vi "Purge.vi"(5 "Digital I/O Pin":u8=7, 7 "Arduino Resource":T1={"VISA resource"="GlueCTRL", "Board Type"=enum."Uno", "Connection Type"=enum."USB / Serial", "Bytes Per Packet (15)"=15}, 9 "Axis Speeds":T3={"X [mm/s]"=25.0, "Y [mm/s]"=25.0, "Z [mm/s]"=10.0}, 10 "Start Position [mm]":dbl[](array[numeric]), 11 ".NET Refnum In":refnum<k24>) -> ()   [LabVIEW 2016]
uses:
  C:/Users/Aerotech/Documents/BNLStaveAssembly-blueprint/Bin/Aerotech.A3200.dll
  BNLStaveAssembly-blueprint/Bin/Aerotech.A3200.dll
  <vilib>/LabVIEW Interface for Arduino/Type Defs/Arduino Resource.ctl
  <vilib>/LabVIEW Interface for Arduino/Type Defs/Board Type.ctl
  <vilib>/LabVIEW Interface for Arduino/LabVIEW Interface for Arduino.lvlib
panel:
  in  "Absolute Purge Height [mm]":dbl=-30.0 format="%#_13g"
  in  "Relative Change in X, Y to Purge [mm]":dbl[](array[numeric])=[0.0, -50.0, 0.0]
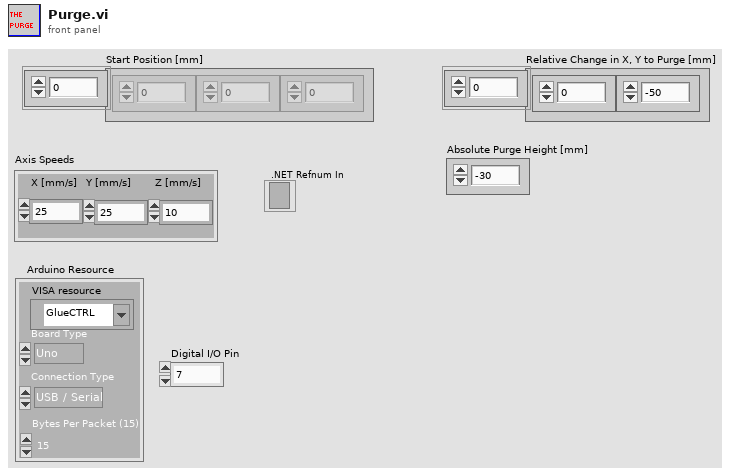
[diagram p1: front panel]
types:
  T1 = typedef "LabVIEW Interface for Arduino.lvlib/Arduino Resource.ctl" = cluster{"VISA resource":refnum<visa-resource-name>, "Board Type":T2, "Connection Type":enum8{"USB / Serial"}, "Bytes Per Packet (15)":u8}
  T2 = typedef "LabVIEW Interface for Arduino.lvlib/Board Type.ctl" = enum16{"Uno", "Dimuelanove w/Atmega 328", "Mega 2560"}
  T3 = cluster{"X [mm/s]":dbl, "Y [mm/s]":dbl, "Z [mm/s]":dbl}
  T4 = cluster{"Start Position [mm][0]":dbl, "Start Position [mm][1]":dbl, "Start Position [mm][2]":dbl}
  T5 = cluster{"Final X":dbl, "Final Y":dbl, "Final Z":dbl}
  T6 = cluster{"Final Position[0]":dbl, "Final Position[1]":dbl, "Final Position[2]":dbl}
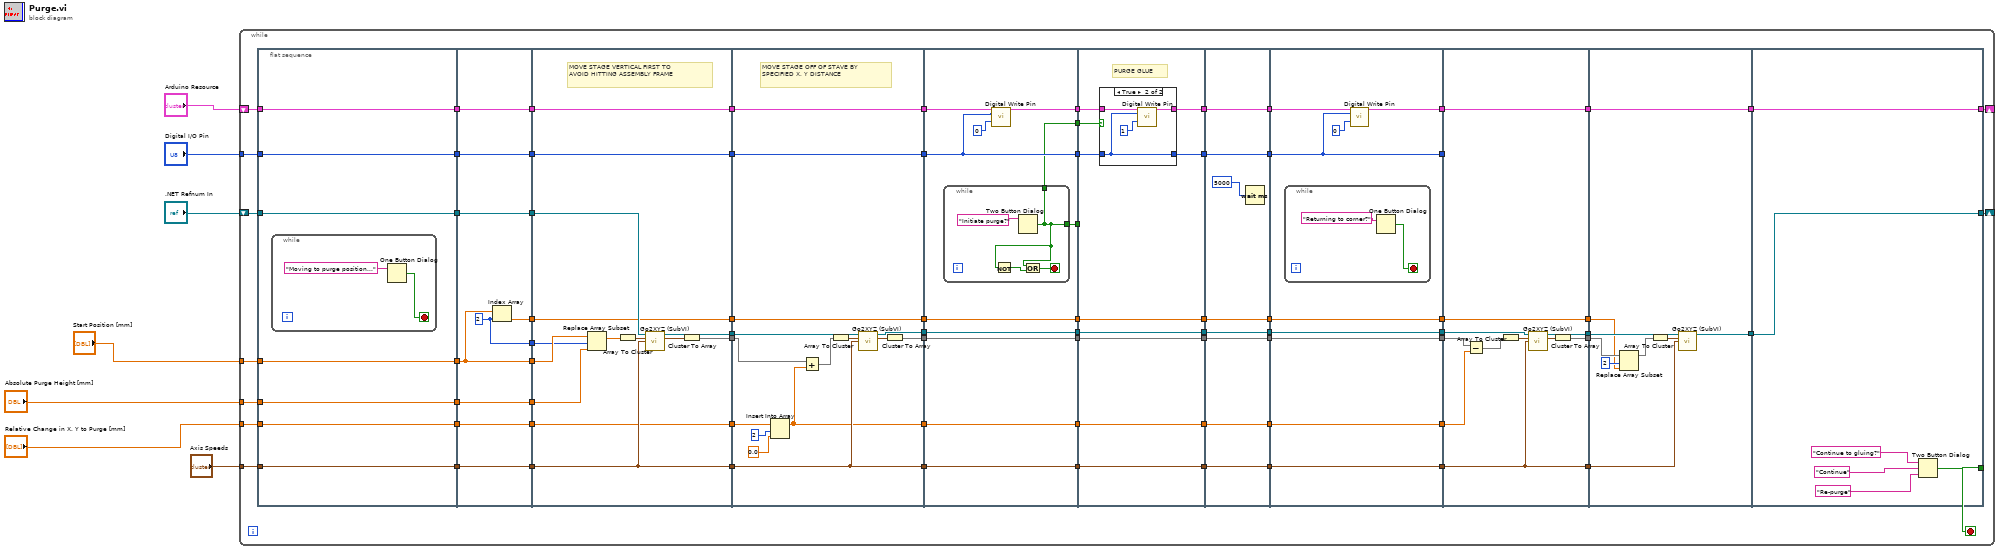
[diagram p0: block diagram]
diagram:
  n1 = while {
    tunnel: "Start Position [mm]" -> [w83]
    tunnel: "Relative Change in X, Y to Purge [mm]" -> [w82]
    tunnel: "Axis Speeds" -> [w81]
    shift-right: [w77] -> _
    shift-left: ".NET Refnum In" -> [w80]
    tunnel: "Digital I/O Pin" -> [w75]
    shift-right: [w70] -> _
    shift-left: "Arduino Resource" -> [w76]
    tunnel: "Absolute Purge Height [mm]" -> [w47]
    stop <- w84 stop-if-true
    n2 = flat-sequence {
      tunnel: [w91] -> w23
      tunnel: w83 -> [w91]
      tunnel: w82 -> [w90]
      tunnel: [w90] -> w21
      tunnel: [w89] -> w19
      tunnel: w81 -> [w89]
      tunnel: [w88] -> w17
      tunnel: w80 -> [w88]
      tunnel: [w87] -> w15
      tunnel: w76 -> [w87]
      tunnel: w75 -> [w86]
      tunnel: [w86] -> w13
      tunnel: w47 -> [w85]
      tunnel: [w85] -> w11
      tunnel: w23 -> [w96]
      tunnel: [w96] -> w22
      tunnel: w21 -> [w102]
      tunnel: [w102] -> w20
      tunnel: w19 -> [w101]
      tunnel: [w101] -> w18
      tunnel: w17 -> [w100]
      tunnel: [w100] -> w16
      tunnel: w15 -> [w99]
      tunnel: [w99] -> w14
      tunnel: w13 -> [w98]
      tunnel: [w98] -> w12
      tunnel: w11 -> [w97]
      tunnel: [w97] -> w10
      tunnel: [w95] -> w9
      tunnel: [w94] -> w8
      tunnel: w22 -> [w105]
      tunnel: w20 -> [w109]
      tunnel: w18 -> [w114]
      tunnel: w16 -> [w116]
      tunnel: [w115] -> w57
      tunnel: [w114] -> w55
      tunnel: w14 -> [w113]
      tunnel: [w113] -> w53
      tunnel: w12 -> [w112]
      tunnel: [w112] -> w51
      tunnel: [w110] -> w49
      tunnel: [w109] -> w48
      tunnel: w10 -> [w107]
      tunnel: [w104] -> w30
      tunnel: w9 -> [w104]
      tunnel: w8 -> [w103]
      tunnel: w57 -> [w129]
      tunnel: [w128] -> w56
      tunnel: w55 -> [w121]
      tunnel: [w121] -> w54
      tunnel: w53 -> [w131]
      tunnel: [w131] -> w52
      tunnel: w51 -> [w130]
      tunnel: [w130] -> w50
      tunnel: w49 -> [w126]
      tunnel: w48 -> [w122]
      tunnel: [w119] -> w46
      tunnel: [w118] -> w33
      tunnel: w30 -> [w117]
      tunnel: [w117] -> w29
      tunnel: [w142] -> w74
      tunnel: w56 -> [w142]
      tunnel: [w141] -> w73
      tunnel: w54 -> [w141]
      tunnel: w52 -> [w139]
      tunnel: w50 -> [w137]
      tunnel: [w138] -> w72
      tunnel: [w137] -> w69
      tunnel: [w136] -> w67
      tunnel: [w135] -> w66
      tunnel: w46 -> [w134]
      tunnel: [w134] -> w38
      tunnel: [w133] -> w34
      tunnel: w33 -> [w133]
      tunnel: w29 -> [w132]
      tunnel: [w132] -> w24
      tunnel: w74 -> [w156]
      tunnel: [w156] -> w65
      tunnel: w73 -> [w155]
      tunnel: [w155] -> w63
      tunnel: w72 -> [w154]
      tunnel: [w153] -> w61
      tunnel: [w151] -> w59
      tunnel: w69 -> [w152]
      tunnel: w67 -> [w150]
      tunnel: w66 -> [_]
      tunnel: [w149] -> w39
      tunnel: w38 -> [w149]
      tunnel: [w148] -> w35
      tunnel: w34 -> [w148]
      tunnel: [w147] -> w25
      tunnel: w24 -> [w147]
      tunnel: w65 -> [w170]
      tunnel: [w170] -> w64
      tunnel: w63 -> [w169]
      tunnel: [w169] -> w62
      tunnel: w61 -> [w168]
      tunnel: [w168] -> w60
      tunnel: w59 -> [w167]
      tunnel: [w167] -> w58
      tunnel: [w165] -> w40
      tunnel: w39 -> [w165]
      tunnel: [w164] -> w36
      tunnel: w35 -> [w164]
      tunnel: [w163] -> w26
      tunnel: w25 -> [w163]
      tunnel: w64 -> [w179]
      tunnel: [w179] -> w79
      tunnel: w62 -> [w178]
      tunnel: [w178] -> w78
      tunnel: w60 -> [w176]
      tunnel: [w175] -> w71
      tunnel: w58 -> [w174]
      tunnel: [w174] -> w68
      tunnel: [w173] -> w41
      tunnel: w40 -> [w173]
      tunnel: [w172] -> w37
      tunnel: w36 -> [w172]
      tunnel: [w171] -> w27
      tunnel: w26 -> [w171]
      tunnel: w79 -> [w191]
      tunnel: w78 -> [w183]
      tunnel: [w190] -> w45
      tunnel: [w189] -> w43
      tunnel: w71 -> [w189]
      tunnel: w68 -> [_]
      tunnel: w41 -> [w188]
      tunnel: w37 -> [w186]
      tunnel: [w184] -> w32
      tunnel: [w183] -> w31
      tunnel: [w182] -> w28
      tunnel: w27 -> [w182]
      tunnel: w45 -> [w200]
      tunnel: [w199] -> w44
      tunnel: w43 -> [w201]
      tunnel: [w201] -> w42
      tunnel: w32 -> [w196]
      tunnel: w31 -> [w197]
      tunnel: w28 -> [w194]
      tunnel: [w206] -> w84
      tunnel: w44 -> [w205]
      tunnel: [w205] -> w77
      tunnel: [w204] -> w70
      tunnel: w42 -> [w204]
      frame #0 {
        n3 = while {
          stop <- w92 stop-if-true
          n4 = One Button Dialog(message="Moving to purge position...") -> (true=w92:bool)  [unwired: 1 in]
        }
      }
      frame #1 {
        w94 = 2 ("index")
        n5 = Index Array(array=w96, index=w94) -> (element=w95:dbl)
      }
      frame #2 {
        # "MOVE STAGE VERTICAL FIRST TO\nAVOID HITTING ASSEMBLY FRAME"
        n6 = Replace Array Subset(array=w105, new element=w107, index=w103) -> (w106:dbl[])
        n7 = Array To Cluster(array=w106) -> (cluster=w108:T4)
        n8 = call "Go2XYZ (SubVI).vi"(".NET Refnum in"=w116, "Go to Coordinates"=w108, "Axis Speeds"=w114) -> (".NET Refnum out"=w115:refnum<k24>, "Final Position"=w111:T5)  [unwired: 8 in, 3 out]
        n9 = Cluster To Array(cluster=w111) -> (array=w110:dbl[])
      }
      frame #3 {
        # "MOVE STAGE OFF OF STAVE BY\nSPECIFIED X, Y DISTANCE"
        n10 = Insert Into Array(array=w122, index=2, new element=0.0 ("new element/subarray")) -> (w118:dbl[])
        n11 = Add(x=w126, y=w118) -> (x+y=w125:dbl[])
        n12 = Array To Cluster(array=w125) -> (cluster=w127:cluster{"[0]":dbl, "[1]":dbl, "[2]":dbl})
        n13 = call "Go2XYZ (SubVI).vi"(".NET Refnum in"=w129, "Go to Coordinates"=w127, "Axis Speeds"=w121) -> (".NET Refnum out"=w128:refnum<k24>, "Final Position"=w120:T5)  [unwired: 8 in, 3 out]
        n14 = Cluster To Array(cluster=w120) -> (array=w119:dbl[])
      }
      frame #4 {
        n15 = while {
          tunnel: [w143] -> w136
          tunnel: [w143] -> w135
          stop <- w144 stop-if-true
          n16 = Two Button Dialog(message="Initiate purge?") -> (T button?=w143:bool)  [unwired: 2 in]
          n17 = Not(x=w143) -> (.not. x?=w145:bool)
          n18 = Or(x=w143, y=w145) -> (x .or. y?=w144:bool)
        }
        n19 = call <vilib>:"Digital Write Pin.vi"("Arduino Resource"=w139, "Digital I/O Pin (0)"=w137, "Value (0)"=u8 0) -> ("Arduino Resource"=w138:T1)  [unwired: 11 in, 1 out]
      }
      frame #5 {
        # "PURGE GLUE"
        n20 = case shown="True" w150 {
          tunnel: w154 -> [w157 w161]
          tunnel: [w157 w160] -> w153
          tunnel: w152 -> [w158 w159]
          tunnel: [w158 w159] -> w151
          frame False {
          }
          frame True {
            n21 = call <vilib>:"Digital Write Pin.vi"("Arduino Resource"=w161, "Digital I/O Pin (0)"=w159, "Value (0)"=u8 1) -> ("Arduino Resource"=w160:T1)  [unwired: 11 in, 1 out]
          }
        }
      }
      frame #6 {
        n22 = Wait (ms)(milliseconds to wait=u32 5000) -> ()  [unwired: 1 out]
      }
      frame #7 {
        n23 = while {
          stop <- w181 stop-if-true
          n24 = One Button Dialog(message="Returning to corner?") -> (true=w181:bool)  [unwired: 1 in]
        }
        n25 = call <vilib>:"Digital Write Pin.vi"("Arduino Resource"=w176, "Digital I/O Pin (0)"=w174, "Value (0)"=u8 0) -> ("Arduino Resource"=w175:T1)  [unwired: 11 in, 1 out]
      }
      frame #8 {
        n26 = Subtract(x=w188, y=w186) -> (x-y=w187:dbl[])
        n27 = Array To Cluster(array=w187) -> (cluster=w192:cluster{"[0]":dbl, "[1]":dbl, "[2]":dbl})
        n28 = call "Go2XYZ (SubVI).vi"(".NET Refnum in"=w191, "Go to Coordinates"=w192, "Axis Speeds"=w183) -> (".NET Refnum out"=w190:refnum<k24>, "Final Position"=w185:T5)  [unwired: 8 in, 3 out]
        n29 = Cluster To Array(cluster=w185) -> (array=w184:dbl[])
      }
      frame #9 {
        n30 = Replace Array Subset(array=w196, new element=w194, index=2) -> (w193:dbl[])
        n31 = Array To Cluster(array=w193) -> (cluster=w198:T6)
        n32 = call "Go2XYZ (SubVI).vi"(".NET Refnum in"=w200, "Go to Coordinates"=w198, "Axis Speeds"=w197) -> (".NET Refnum out"=w199:refnum<k24>)  [unwired: 8 in, 4 out]
      }
      frame #10 {
        n33 = Two Button Dialog(message="Continue to gluing?", 1:"Re-purge" ("F button name (\"Cancel\")"), 2:"Continue" ("T button name (\"OK\")")) -> (T button?=w206:bool)
      }
    }
  }
